vi "dbc-close-frame-tag.vi"(8 "error in (no error)":errorcluster, 11 "dbc in":refnum<class "dbc.lvclass">) -> (0 "error out":errorcluster, 3 "dbc out":refnum<class "dbc.lvclass">)   [LabVIEW 2015, in "dbc.lvclass"]
uses:
  dbc.lvclass
  dbc.lvclass/dbc.ctl
  Read-active-frame-tag.vi
  Write-active-frame-tag.vi
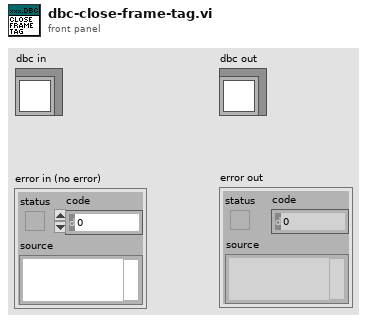
[diagram p1: front panel]
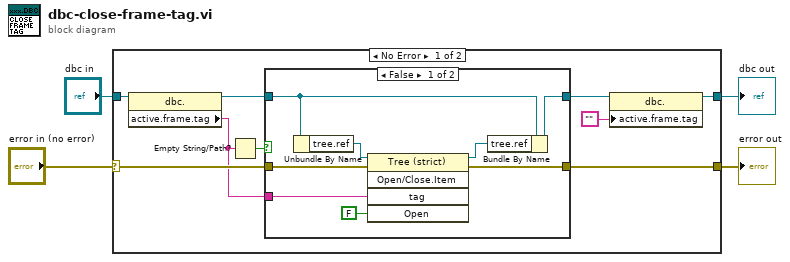
[diagram p0: block diagram]
diagram:
  n1 = case shown="No Error" "error in (no error)" {
    selector: "error in (no error)" -> [w10 w25]
    tunnel: [w12 w25] -> w3
    tunnel: [w6 w24] -> w1
    tunnel: "dbc in" -> [w13 w24]
    frame No Error {
      n2 = property class="dbc."(reference=w13) -> (reference out=w9:refnum<class "dbc.lvclass">, "active.frame.tag"=w7:string)  [unwired: 1 in, 1 out]
      n3 = Empty String/Path?(string/path=w7) -> (empty?=w8:bool)
      n4 = case shown="False" w8 {
        tunnel: [w20 w22] -> w12
        tunnel: [w19 w23] -> w11
        tunnel: w10 -> [w17 w22]
        tunnel: w9 -> [w15 w23]
        tunnel: w7 -> [w14 _]
        frame False {
          n5 = Unbundle By Name(w15) -> ("tree.ref"=w16:refnum<vi>)
          n6 = invoke class="Tree (strict)" method="Open/Close.Item"(reference=w16, error in=w17, "tag"=w14, "Open"=FALSE ("Open?")) -> (reference out=w18:refnum<vi>, error out=w20:errorcluster)  [unwired: 1 in, 3 out]
          n7 = Bundle By Name(cluster=w15, "tree.ref"=w18) -> (w19:refnum<class "dbc.lvclass">)
        }
        frame True {
        }
      }
      n8 = property class="dbc."(reference=w11, "active.frame.tag"="") -> (reference out=w6:refnum<class "dbc.lvclass">)  [unwired: 1 in, 1 out]
    }
    frame Error {
    }
  }
  "error out" <- w3
  "dbc out" <- w1
